vi "Stop Module.vi"(8 "error in":errorcluster) -> (0 "error out":errorcluster)   [LabVIEW 2014, in "Events Lib.lvlib"]
uses:
  Events Lib.lvlib
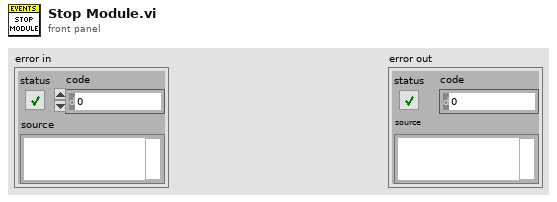
[diagram p1: front panel]
types:
  T1 = enum16{"Create Events", "Get Events", "Destroy Events"}
  T2 = typedef "Events Lib.lvlib/Events TypeDef.ctl" = cluster{"Stop Event":refnum<user-event>, "Chart Send Value":refnum<user-event>, "Show Module":refnum<user-event>, "Hide Module":refnum<user-event>}
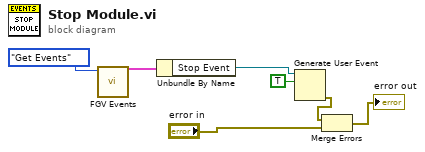
[diagram p0: block diagram]
diagram:
  n1 = call "FGV Events.vi"("Action"=T1."Get Events") -> ("Cluster"=w3:T2)  [unwired: 9 in, 1 out]
  n2 = Unbundle By Name(w3) -> ("Stop Event"=w2:refnum<user-event>)
  n3 = Generate User Event(user event=w2, event data cluster=TRUE ("event data")) -> (error out=w7:errorcluster)  [unwired: 2 in, 1 out]
  n4 = Merge Errors(w7, "error in") -> (→"error out":errorcluster)
